vi "DIO_Test.vi"() -> ()   [LabVIEW 2019]
uses:
  <vilib>/rvi/interface/nirviOpenFPGA/nirviOpenFPGA.xnode
  LVMQTT-master/MQTT_Functions.lvlib
  LVMQTT-master/Controls/Retain_Flag.ctl
  LVMQTT-master/Controls/DUP_Flag.ctl
  LVMQTT-master/Controls/QoS.ctl
  LVMQTT-master/Controls/Connect_Flags.ctl
  <vilib>/rvi/interface/nirviReadWriteControl/nirviReadWriteControl.xnode
  FPGA Bitfiles/sbrio-9642sauna_FPGATarget_FPGAMAin_1KjVu7nH5Fw.lvbitx
  FPGA_MAin.vi
  <vilib>/FPGAPlugInAG/cRIO-9068/niLvFpga_Open_cRIO-9068.vi
  <vilib>/rvi/interface/common/dynamic/niFpgaDynamicAddResources.vi
  NiFpgaLv.dll
  <vilib>/Utility/error.llb/Error Cluster From Error Code.vi
  <vilib>/rvi/interface/Simulation/niFpgaSimulationCallBeginRW.vi
  <vilib>/rvi/errors/niLvFpgaAdjustHostInterfaceError.vi
  LVMQTT-master/Controls/Connection_Return_Codes.ctl
panel:
  out "value":T1
  out "Message":string
  in  "Client ID":string="LVSubscribeClient"
  in  "Stop Reading":bool
  out "Granted QoS Levels":T2[](array[typedef])
  out "Connection Status":T3=enum."Connection refused: Server unavailable"
  out "error out":errorcluster
  in  "error in (no error)":errorcluster
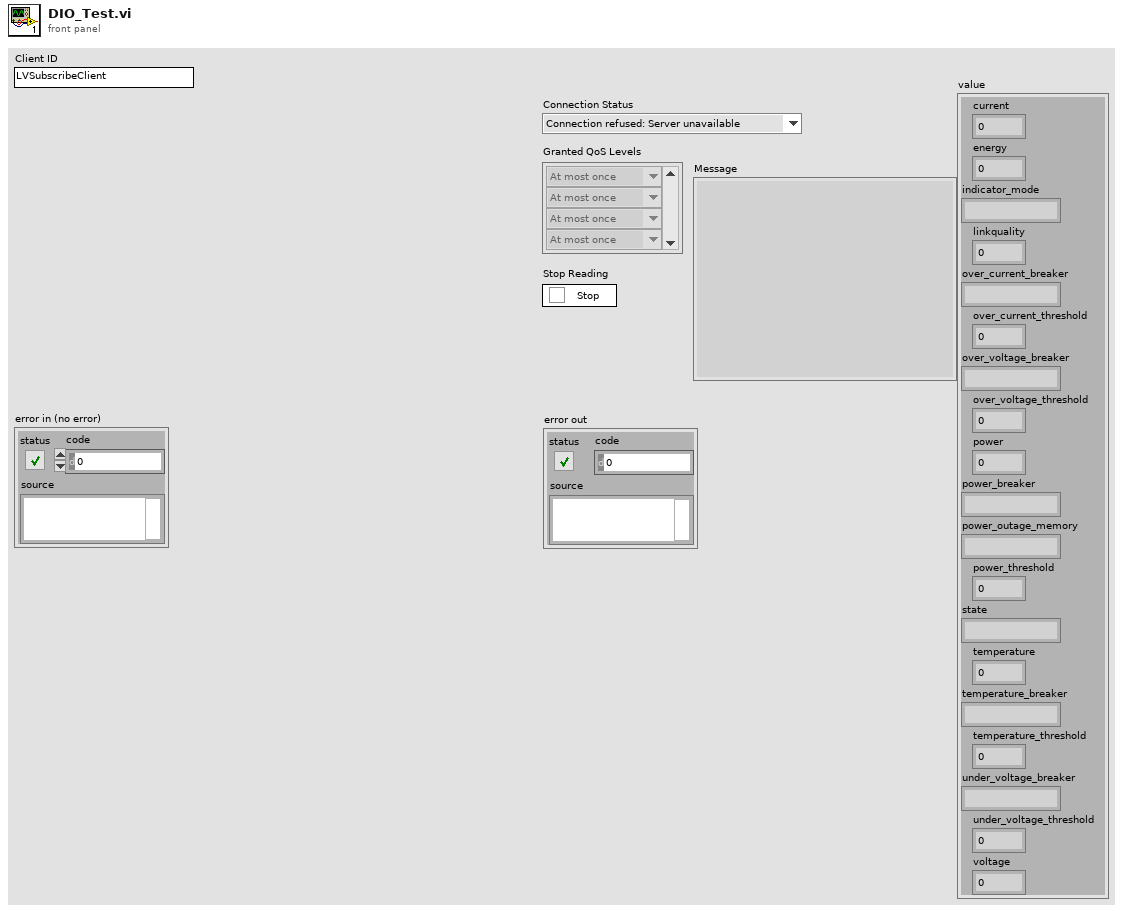
[diagram p1: front panel]
types:
  T1 = cluster{"current":dbl, "energy":dbl, "indicator_mode":string, "linkquality":i32, "over_current_breaker":string, "over_current_threshold":dbl, "over_voltage_breaker":string, "over_voltage_threshold":dbl, "power":dbl, "power_breaker":string, "power_outage_memory":string, "power_threshold":dbl, "state":string, "temperature":dbl, "temperature_breaker":string, "temperature_threshold":dbl, "under_voltage_breaker":string, "under_voltage_threshold":dbl, "voltage":dbl}
  T2 = typedef "MQTT_Functions.lvlib/QoS.ctl" = enum8{"At most once", "At least once", "Exactly once", "Reserved"}
  T3 = typedef "MQTT_Functions.lvlib/Connection_Return_Codes.ctl" = enum16{"Connection accepted", "Connection refused: unacceptable protocol version", "Connection refused: identifier rejected", "Connection refused: Server unavailable", "Connection refused: bad user name or password", "Connection refused: not authorized"}
  T4 = typedef "MQTT_Functions.lvlib/Connect_Flags.ctl" = cluster{"user name":bool, "password":bool, "will retain":bool, "will flag":bool, "clean session":bool, "reserved":bool, "will QoS":T2}
  T5 = typedef "MQTT_Functions.lvlib/DUP_Flag.ctl" = bool
  T6 = typedef "MQTT_Functions.lvlib/Retain_Flag.ctl" = bool
  T7 = cluster{"QoS":T2, "DUP":T5, "Retain":T6, "Keep Alive (sec)":u16}
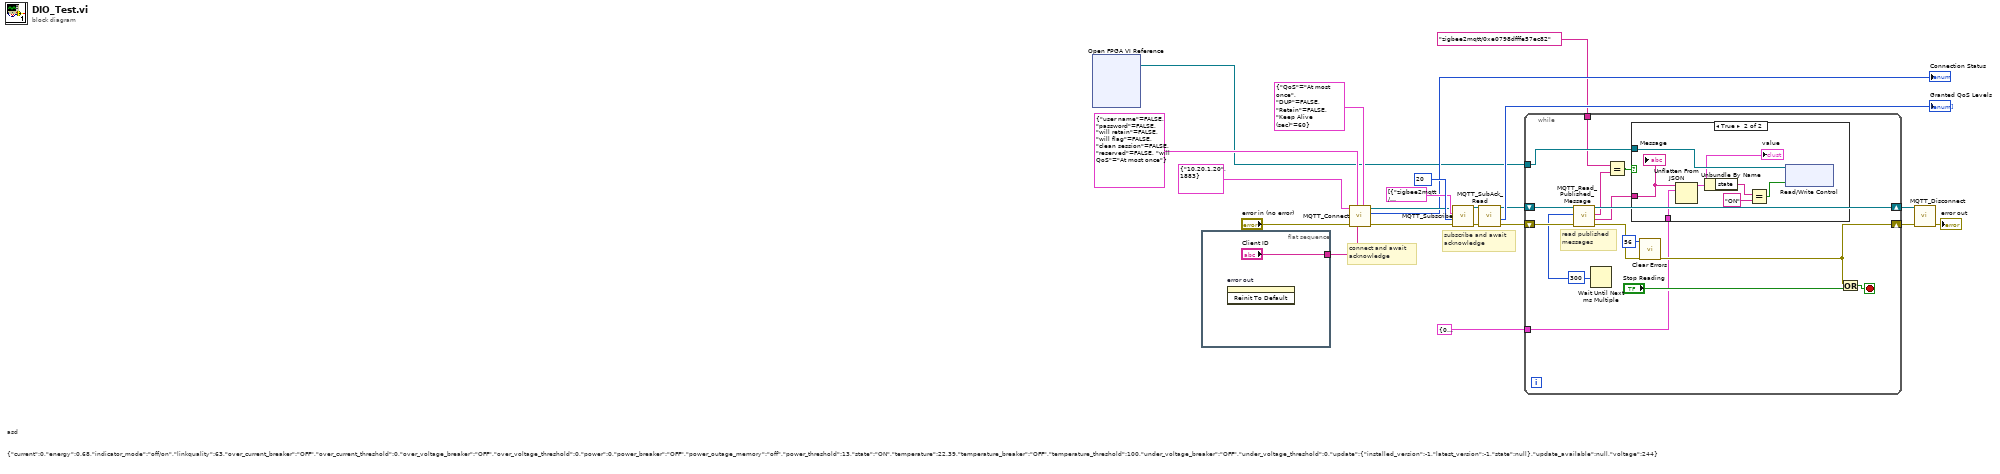
[diagram p0: block diagram]
diagram:
  # "asd\n\n\n{\"current\":0,\"energy\":0.68,\"indicator_mode\":\"off/on\",\"linkquality\":63,\"over_current_breaker\":\"OFF\",\"over_current_threshold\":0,\"over_voltage_breaker\":\"OFF\",\"over_voltage_threshold\":0,\"power\":0,\"power_breaker\":\"OFF\",\"power_outage_memory\":\"off\",\"power_threshold\":13,\"state\":\"ON\",\"temperature\":22.39,\"temperature_breaker\":\"OFF\",\"temperature_threshold\":100,\"under_voltage_breaker\":\"OFF\",\"under_voltage_threshold\":0,\"update\":{\"installed_version\":-1,\"latest_version\":-1,\"state\":null},\"update_available\":null,\"voltage\":244}"
  # "connect and await\nacknowledge"
  # "subscribe and await\nacknowledge"
  n1 = xnode "Open FPGA VI Reference"() -> ("FPGA VI Reference Out"=w3:refnum<k20>)  [unwired: 2 in, 1 out]
  n2 = flat-sequence {
    tunnel: ["Client ID"] -> w21
    frame #0 {
      n3 = invoke on="error out" class="Clust (strict)" method="Reinit To Default"() -> ()  [unwired: 3 in, 3 out]
    }
  }
  n4 = call "MQTT_Connect.vi"("Connect Meta"=T7 {"QoS"=enum."At most once", "DUP"=FALSE, "Retain"=FALSE, "Keep Alive (sec)"=60}, "Client ID"=w21, "Connect Flags"=T4 {"user name"=FALSE, "password"=FALSE, "will retain"=FALSE, "will flag"=FALSE, "clean session"=FALSE, "reserved"=FALSE, "will QoS"=enum."At most once"}, "error in (no error)"="error in (no error)", "MQTT Broker"=cluster{"address (IP)":string, "port":u16} {"address (IP)"="10.20.1.20", "port"=1883}) -> ("error out"=w4:errorcluster, "Connection Status"=→"Connection Status":T3, "connection ID out"=w6:refnum<k5>)  [unwired: 4 in]
  n5 = call "MQTT_Subscribe.vi"("error in (no error)"=w4, "Message ID"=u16 20, "Subscription Info Array"=cluster{"Topic":string, "QoS":T2}[] [{"Topic"="zigbee2mqtt/0xe0798dfffe57ec82", "QoS"=enum."At most once"}], "connection ID"=w6) -> ("error out"=w14:errorcluster, "connection ID out"=w15:refnum<k5>)  [unwired: 6 in]
  n6 = call "MQTT_SubAck_Read.vi"("error in (no error)"=w14, "connection ID"=w15) -> ("error out"=w12:errorcluster, "Granted QoS Levels"=→"Granted QoS Levels":T2[], "connection ID out"=w11:refnum<k5>)  [unwired: 7 in]
  n7 = while {
    shift-right: [w30] -> w9
    shift-left: w12 -> [w37]
    shift-right: [w35] -> w10
    shift-left: w11 -> [w36]
    tunnel: w3 -> [w27]
    tunnel: "zigbee2mqtt/0xe0798dfffe57ec82" ("Topic") -> [w26]
    tunnel: T1 {"current"=0.0, "energy"=0.0, "indicator_mode"="", "linkquality"=0, "over_current_breaker"="", "over_current_threshold"=0.0, "over_voltage_breaker"="", "over_voltage_threshold"=0.0, "power"=0.0, "power_breaker"="", "power_outage_memory"="", "power_threshold"=0.0, "state"="", "temperature"=0.0, "temperature_breaker"="", "temperature_threshold"=0.0, "under_voltage_breaker"="", "under_voltage_threshold"=0.0, "voltage"=0.0} ("input cluster") -> [w23]
    stop <- w33 stop-if-true
    w28 = u32 300 ("millisecond multiple")
    # "read published\nmessages"
    n8 = call "MQTT_Read_Published_Message.vi"("error in (no error)"=w37, "timeout ms (25000)"=w28, "connection ID"=w36) -> ("error out"=w29:errorcluster, "Message"=w34:string, "Topic Name"=w25:string, "connection ID out"=w35:refnum<k5>)  [unwired: 3 in, 2 out]
    n9 = Wait Until Next ms Multiple(millisecond multiple=w28) -> ()  [unwired: 1 out]
    n10 = Equal?(x=w26, y=w25) -> (x = y?=w24:bool)
    n11 = case shown="True" w24 {
      tunnel: w34 -> [_ w44]
      tunnel: w27 -> [_ w43]
      tunnel: w23 -> [_ w38]
      frame False {
      }
      frame True {
        n12 = Unflatten From JSON(JSON string=w44, type and defaults=w38) -> (value=w39:T1)  [unwired: 5 in, 1 out]
        "value" <- w39
        n13 = Unbundle By Name(w39) -> ("state"=w42:string)
        n14 = Equal?(x=w42, y="ON") -> (x = y?=w40:bool)
        n15 = xnode "Read/Write Control"("FPGA VI Reference In"=w43, "Kiuas LED"=w40) -> ()  [unwired: 1 in, 2 out]
        "Message" <- w44
      }
    }
    n16 = call <vilib>:"Clear Errors.vi"("error in (no error)"=w29, "specific error code to clear (0: all)"=56) -> ("error out"=w30:errorcluster)  [unwired: 4 in, 1 out]
    n17 = Or(x=w30, y="Stop Reading") -> (x .or. y?=w33:bool)
  }
  n18 = call "MQTT_Disconnect.vi"("error in (no error)"=w9, "connection ID"=w10) -> ("error out"=→"error out":errorcluster)  [unwired: 9 in]
